vi "API_SeperateLayersPython.vi"(6 "Timeout (ms)":u32, 7 "Wait (F)":bool, 8 "error in (no error)":errorcluster, 10 "?":T1, 11 "DLP2 in":refnum<class "DLP2.lvclass">) -> (0 "error out":errorcluster, 2 "targetMaterials":string[](array[string]), 3 "DLP2 out":refnum<class "DLP2.lvclass">)   [LabVIEW 2022 SP3, in "DLP2.lvclass"]
doc: "Developed by Kevin Thompson\nkevin@thompsonengineering.net\n\nCopyright 2018\nThompson Engineering, LLC"
uses:
  DLP2.lvclass
  DataTypes/SeperateLayersPython--cluster.ctl
  Common/Controls/PythonVersion--Enum.ctl
  DataTypes/AsynCmd_Temp01--enum.ctl
  DLP2.lvclass/DLP2.ctl
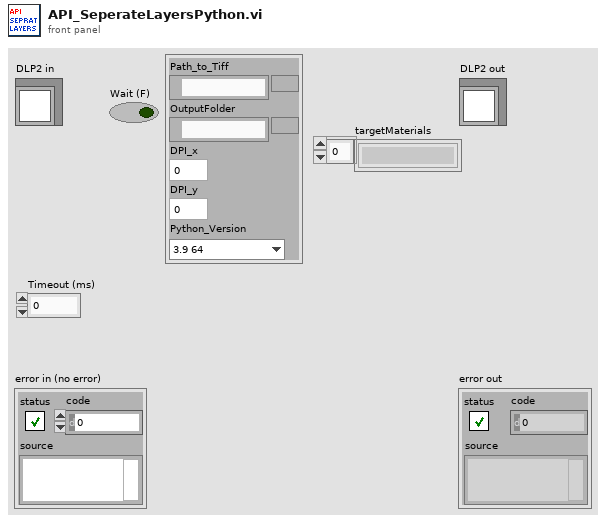
[diagram p1: front panel]
types:
  T1 = typedef "SeperateLayersPython--cluster.ctl" = cluster{"Path_to_Tiff":path, "OutputFolder":path, "DPI_x":i32, "DPI_y":i32, "Python_Version":T2}
  T2 = typedef "PythonVersion--Enum.ctl" = enum16{"3.9 64", "3.9 32", "3.12 64", "3.12 32"}
  T3 = typedef "DLP2.lvclass/AsynCmd_Temp01--enum.ctl" = enum16{"LoadTiffImage", "SeperateLayersPython", "InvokePPP"}
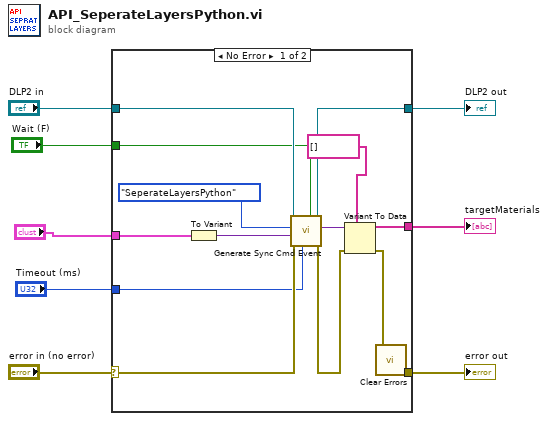
[diagram p0: block diagram]
diagram:
  n1 = case shown="No Error" "error in (no error)" {
    selector: "error in (no error)" -> [w20 w24]
    tunnel: [w9 w24] -> w7
    tunnel: [w21 w23] -> w5
    tunnel: "DLP2 in" -> [w22 w23]
    tunnel: "?" -> [w18 _]
    tunnel: "Wait (F)" -> [w16 _]
    tunnel: "Timeout (ms)" -> [w15 _]
    tunnel: [w11 _] -> w1
    frame No Error {
      n2 = To Variant(anything=w18) -> (Variant=w17:variant)
      n3 = call "Generate Sync Cmd Event.vi"("Wait (F)"=w16, "Timeout (ms)"=w15, "error in (no error)"=w20, "vData"=w17, "AsyncCmd"=AsynCmd_Temp01--enum."SeperateLayersPython", "DLP2 in"=w22) -> ("error out"=w13:errorcluster, "Return Value"=w14:variant, "DLP2 out"=w21:refnum<class "DLP2.lvclass">)  [unwired: 3 in]
      n4 = Variant To Data(error in=w13, type=string[] [] ("targetMaterials"), Variant=w14) -> (data=w11:string[], error out=w12:errorcluster)
      n5 = call <vilib>:"Clear Errors.vi"("error in (no error)"=w12) -> ("error out"=w9:errorcluster)  [unwired: 5 in, 1 out]
    }
    frame Error {
    }
  }
  "error out" <- w7
  "DLP2 out" <- w5
  "targetMaterials" <- w1
